vi "Query Modulation Format Test Pattern.vi"(8 "error in (no error)":errorcluster {"code" format="%.0x"}, 11 "instrument handle":refnum<k15>) -> (0 "error out":errorcluster {"code" format="%.0x"}, 1 "TestPattern":i32, 2 "ModulationType":i32, 3 "instrument handle out":refnum<k15>)   [LabVIEW 2009, in "Keysight XSAn.lvlib"]
doc: "Query modulation format test pattern.\n\nSupported Models: M8920A, M9410A."
uses:
  <instrlib>/Keysight XSAn/Keysight XSAn.lvlib
  AgXSAn.dll
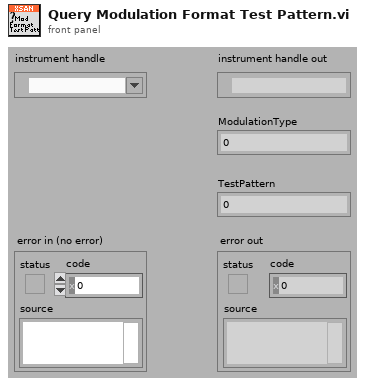
[diagram p1: front panel]
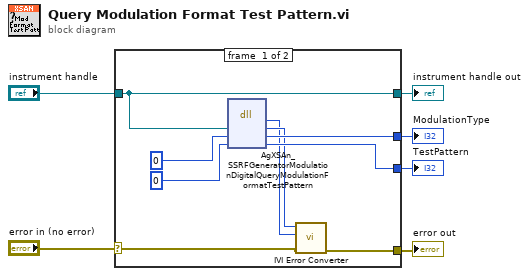
[diagram p0: block diagram]
diagram:
  n1 = case shown="No Error" "error in (no error)" {
    selector: "error in (no error)" -> [w11 w17]
    tunnel: [w10 w17] -> w6
    tunnel: "instrument handle" -> [w7 w16]
    tunnel: [w14 _] -> w3
    tunnel: [w12 _] -> w2
    tunnel: [w7 w16] -> w1
    frame #0 {
      n2 = dll-call lib="AgXSAn**.dll" fn="AgXSAn_SSRFGeneratorModulationDigitalQueryModulationFormatTestPattern"("Vi"=w7, "ModulationType"=0, "TestPattern"=0) -> (w8:i32, "Vi"=w9:u32, "ModulationType"=w14:i32, "TestPattern"=w12:i32)  [unwired: 3 in, 2 out]
      n3 = call <instrlib>:"IVI Error Converter.vi"("error in (no error)"=w11, "IVI error code (0)"=w8, "instrument handle"=w9) -> ("error out"=w10:errorcluster)  [unwired: 7 in, 1 out]
    }
    frame #1 {
    }
  }
  "error out" <- w6
  "instrument handle out" <- w1
  "ModulationType" <- w3
  "TestPattern" <- w2
